vi "字符串入队列操作.vi"(7 "优先插入？":bool, 8 "字符消息入队列":string, 9 "数值":i32, 10 "布尔":bool, 11 "界面切换队列":refnum<queue>) -> (3 "队列输出":refnum<queue>)   [LabVIEW 2018]
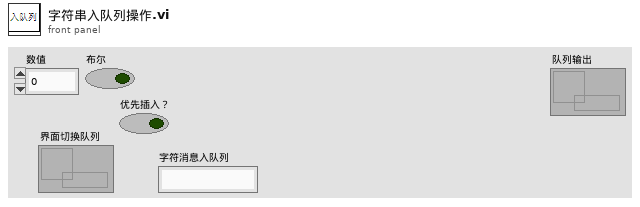
[diagram p1: front panel]
types:
  T1 = typedef "数据簇.ctl" = cluster{"字符串":string, "数值":i32, "布尔":bool}
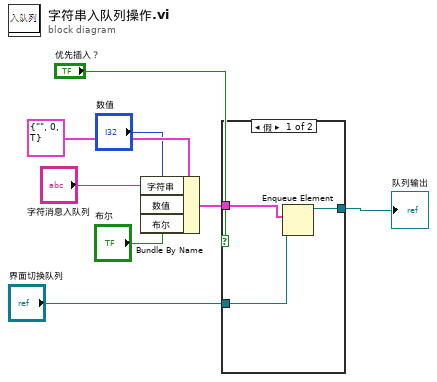
[diagram p0: block diagram]
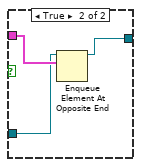
[diagram p2: hidden frame]
diagram:
  n1 = Bundle By Name(cluster=T1 {"字符串"="", "数值"=0, "布尔"=TRUE}, "字符串"="字符消息入队列", "数值"="数值", "布尔"="布尔") -> (w5:T1)
  n2 = case shown="假" "优先插入？" {
    tunnel: "界面切换队列" -> [w11 w13]
    tunnel: w5 -> [w10 w14]
    tunnel: [w9 w12] -> w2
    frame False {
      n3 = Enqueue Element(queue=w11, element=w10) -> (queue out=w9:refnum<queue>)  [unwired: 2 in, 2 out]
    }
    frame True {
      n4 = Enqueue Element At Opposite End(queue=w13, element=w14) -> (queue out=w12:refnum<queue>)  [unwired: 2 in, 2 out]
    }
  }
  "队列输出" <- w2
